vi "scripting build FXP VIs.vi"() -> ()   [LabVIEW 2020]
uses:
  <vilib>/numeric/LVNumericRepresentation.ctl
  <vilib>/Utility/traverseref.llb/TRef TravTarget.ctl
  <vilib>/Utility/traverseref.llb/VI Scripting - Traverse.lvlib
panel:
  out "error out 4":errorcluster
  out "Traverse All":string[][](table)
  out "error out 3":errorcluster
  in  "Array Ref.":refnum<vi>
  in  "Representation":T1(ring)
  in  "error in (no error)":errorcluster
  out "Ref. Out":refnum<vi>
  out "error out":errorcluster
  out "error out 2":errorcluster
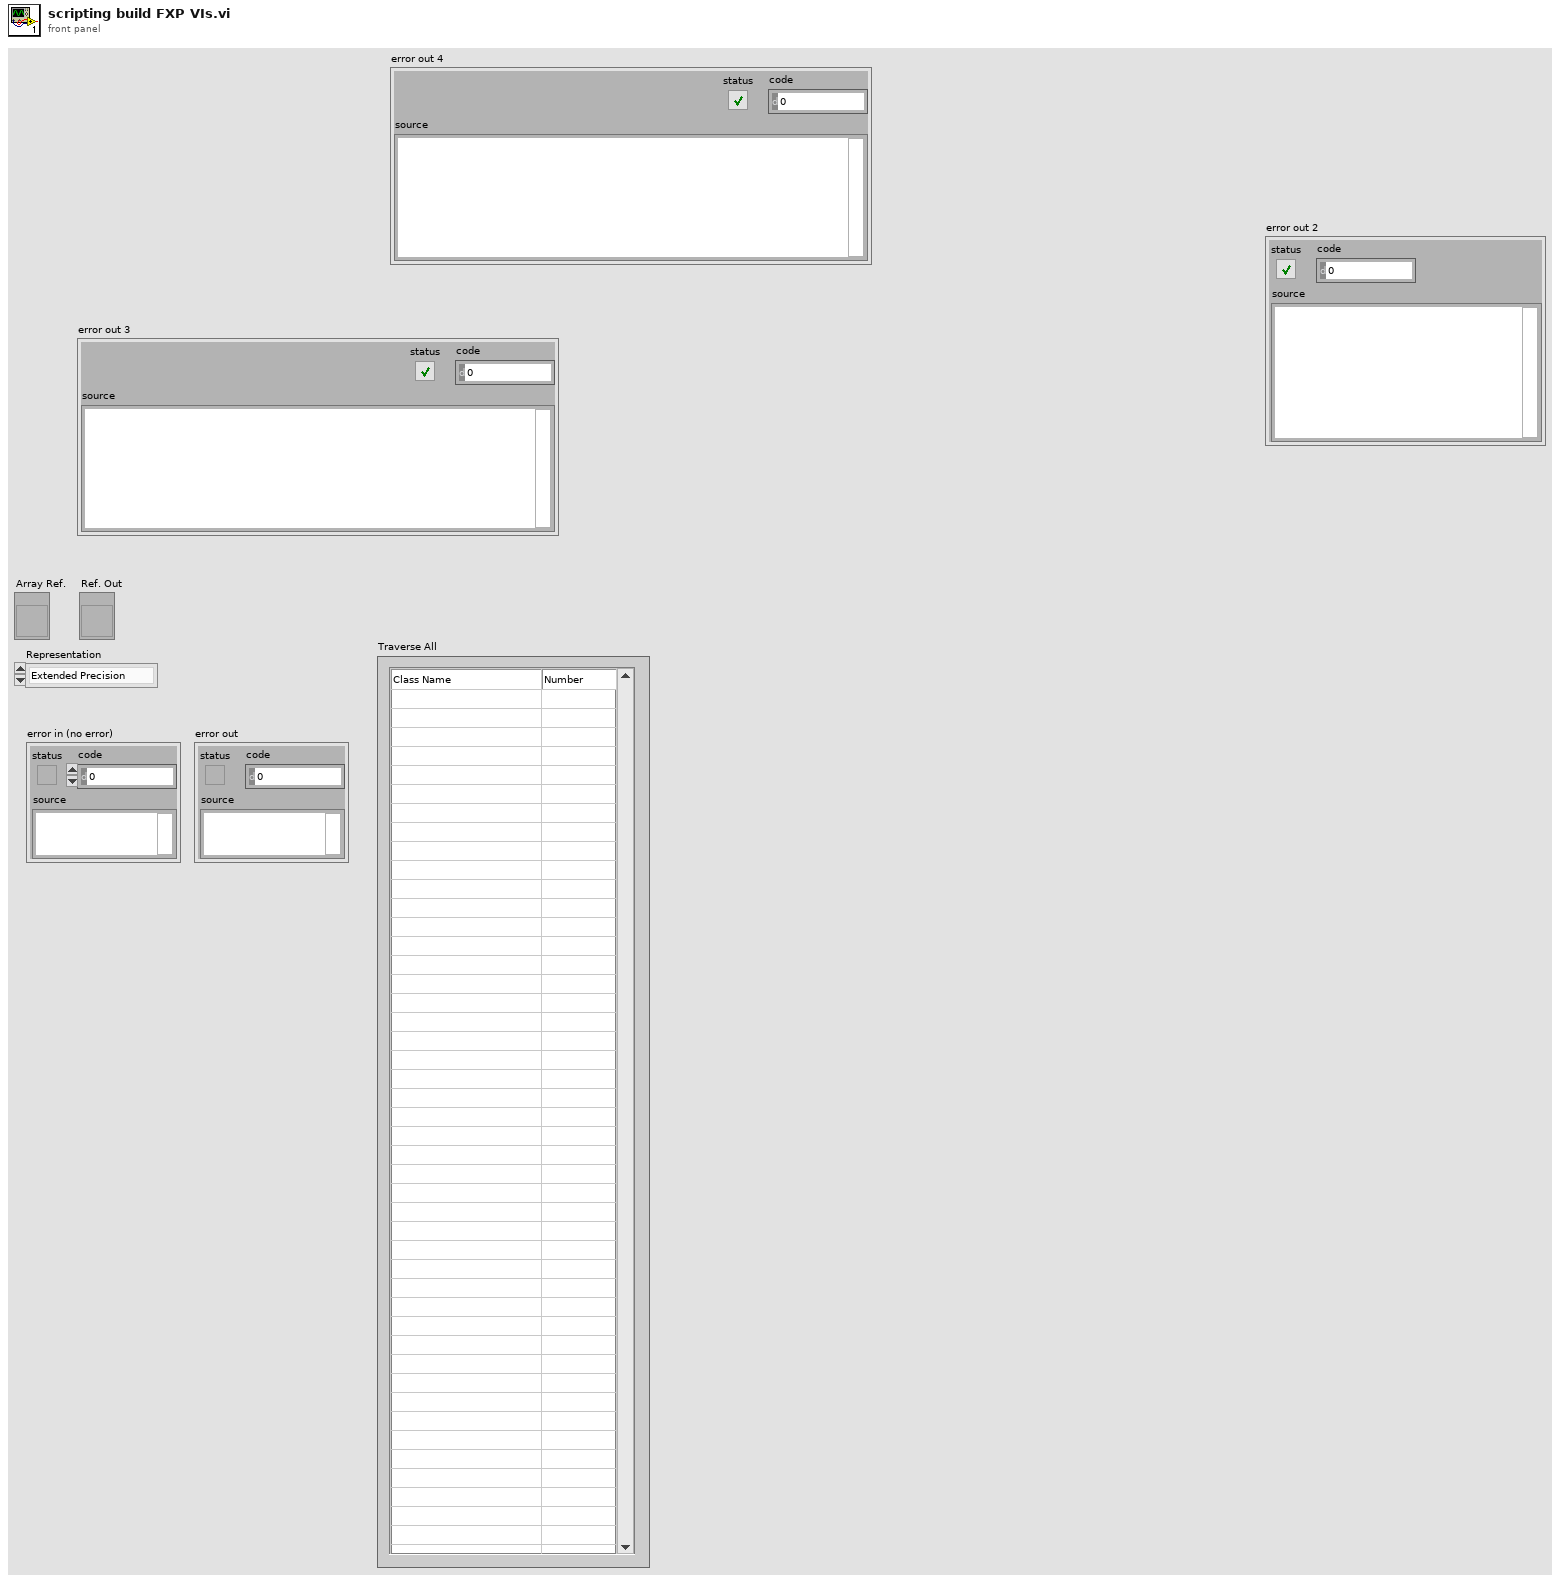
[diagram p1: front panel]
types:
  T1 = enum32{"Extended Precision", "Double Precision", "Single Precision", "Long", "Word", "Byte", "Unsigned Long", "Unsigned Word", "Unsigned Byte", "Complex Extended", "Complex Double", "Complex Single", "Quad", "Unsigned Quad", "Fixed-Point"}
  T2 = typedef "TRef TravTarget.ctl" = enum16{"FP", "BD", "Other"}
  T3 = typedef "LVNumericRepresentation.ctl" = enum32{"Extended Precision", "Double Precision", "Single Precision", "Long", "Word", "Byte", "Unsigned Long", "Unsigned Word", "Unsigned Byte", "Complex Extended", "Complex Double", "Complex Single", "Quad", "Unsigned Quad", "Fixed-Point"}
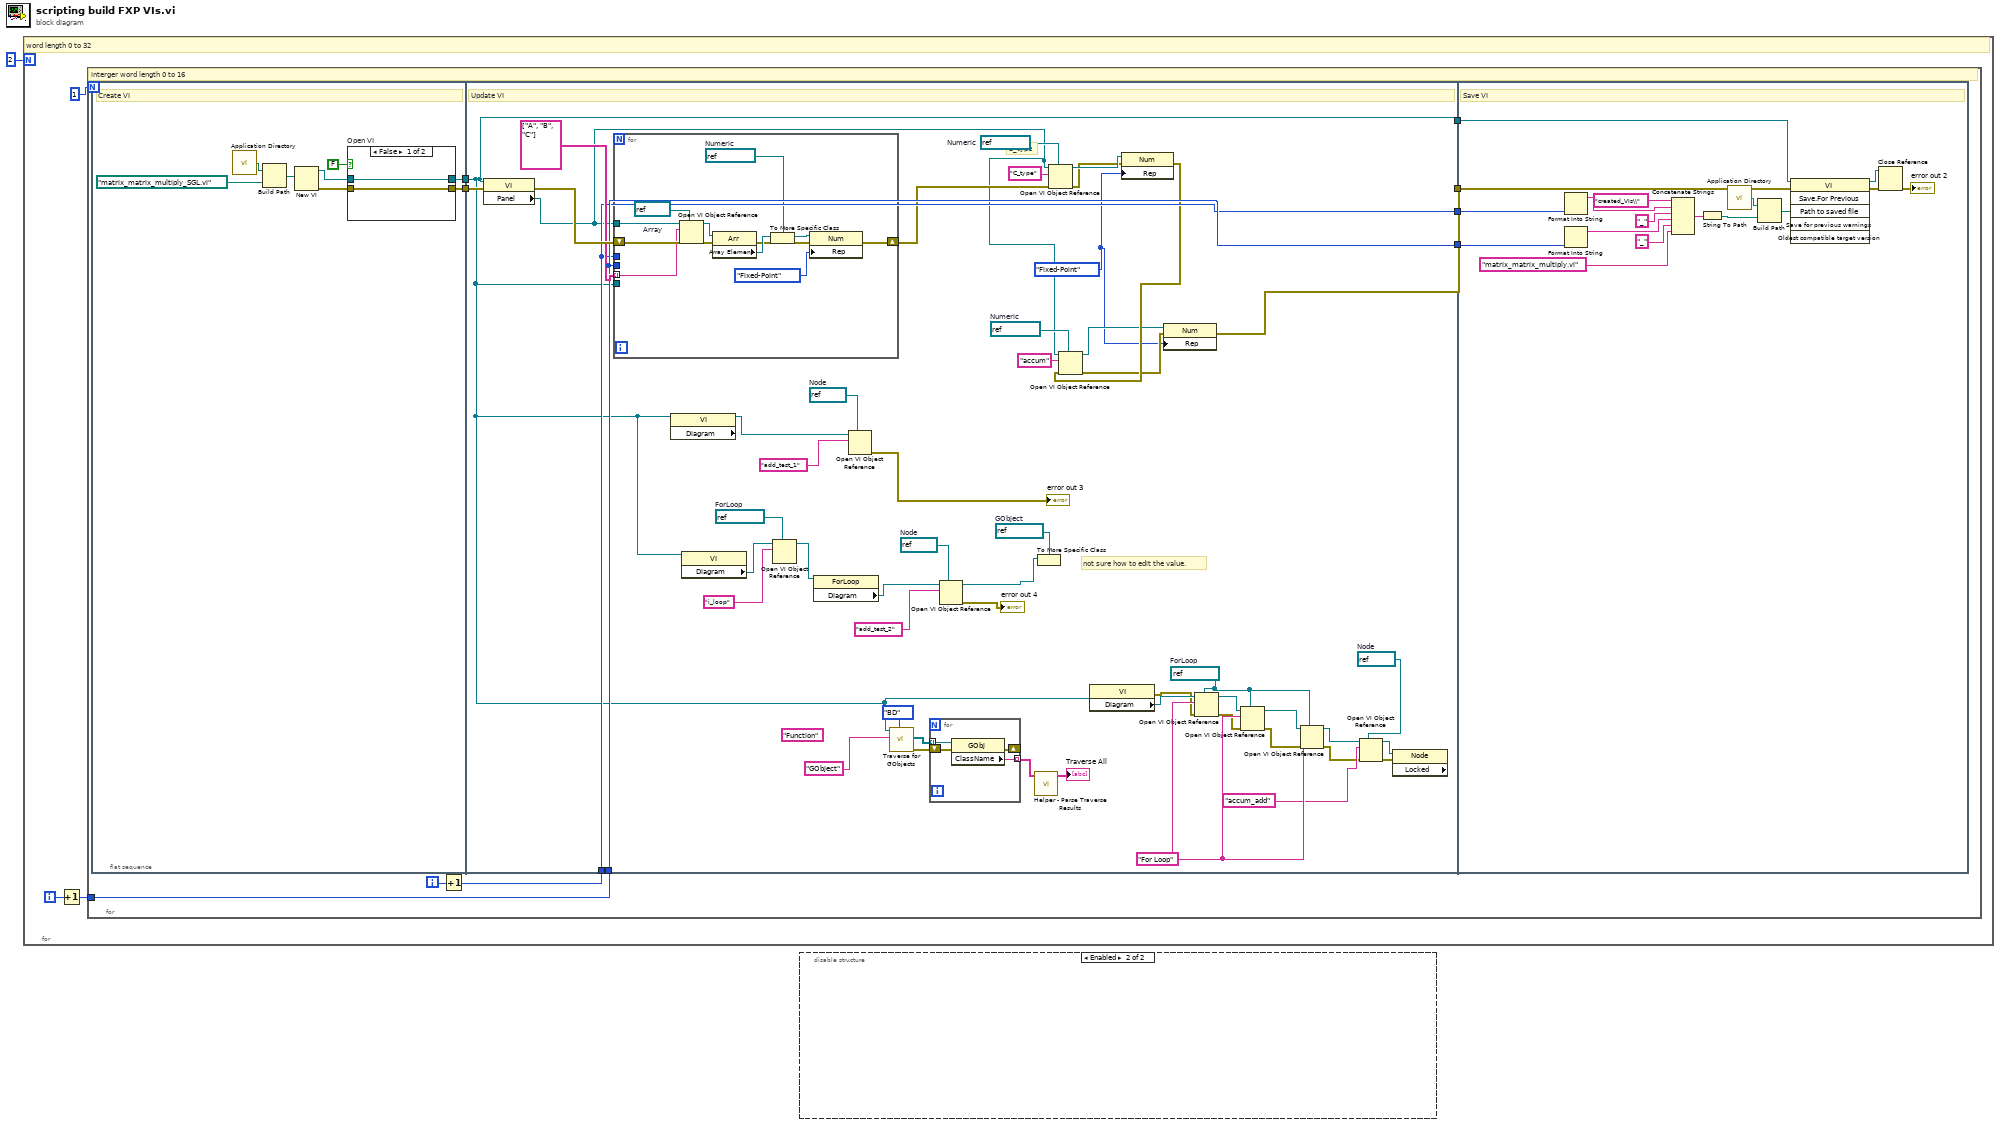
[diagram p0: block diagram]
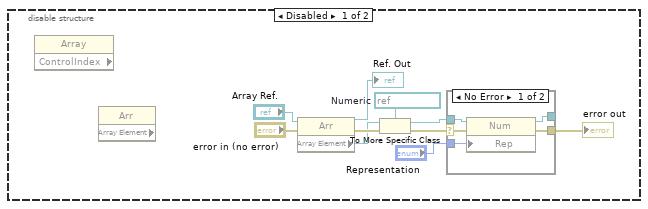
[diagram p2: hidden frame]
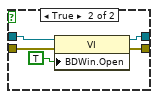
[diagram p4: hidden frame]
diagram:
  n1 = for {
    N: 2 -> [_]
    i -> [w4]
    # "word length 0 to 32"
    n2 = Increment(x=w4) -> (x+1=w2:i32)
    n3 = for {
      N: 1 -> [_]
      tunnel: w2 -> [w7]
      i -> [w6]
      # "interger word length 0 to 16"
      n4 = flat-sequence {
        tunnel: [w14] -> w13
        tunnel: [w15] -> w12
        tunnel: w5 -> [w77]
        tunnel: w7 -> [w78]
        tunnel: w13 -> [w35]
        tunnel: w12 -> [w79]
        tunnel: [w67] -> w11
        tunnel: [w78] -> w10
        tunnel: [w77] -> w9
        tunnel: [w35] -> w8
        tunnel: w11 -> [w103]
        tunnel: w10 -> [w101]
        tunnel: w9 -> [w100]
        tunnel: w8 -> [w99]
        frame #0 {
          # "Create VI"
          n5 = call <vilib>:"Application Directory.vi"() -> ("Application Directory"=w20:path)
          n6 = Build Path(base path=w20, name or relative path=path "matrix_matrix_multiply_SGL.vi" ("vi path")) -> (appended path=w21:path)
          n7 = New VI(10:w21) -> (0:w19:errorcluster, 3:w18:refnum<vi>)  [unwired: 6 in]
          n8 = case "Open VI" shown="False" FALSE {
            tunnel: w18 -> [w22 w28]
            tunnel: w19 -> [w23 w27]
            tunnel: [w22 w25] -> w14
            tunnel: [w23 w24] -> w15
            frame False {
            }
            frame True {
              n9 = property class="VI"(reference=w28, error in=w27, "BDWin.Open"=TRUE ("Block Diagram Window:Open")) -> (reference out=w25:refnum<vi>, error out=w24:errorcluster)
            }
          }
        }
        frame #1 {
          w29 = refnum<vi> refnum  # GObject
          w36 = refnum<vi> refnum  # ForLoop
          w40 = refnum<vi> refnum  # Node
          w49 = refnum<vi> refnum  # Node
          w50 = "For Loop" ("name/order")
          w51 = refnum<vi> refnum  # ForLoop
          (unwired) "Function"
          w63 = refnum<vi> refnum  # Node
          w71 = refnum<vi> refnum  # Numeric
          w64 = LVNumericRepresentation."Fixed-Point" ("Representation")
          w76 = refnum<vi> refnum  # Numeric
          # "not sure how to edit the value."
          # "C_type"
          # "Update VI"
          n10 = property on="Property Node" class="VI"(reference=w35, error in=w79) -> (error out=w81:errorcluster, "Panel"=w69:refnum<vi>)  [unwired: 1 out]
          n11 = for {
            tunnel: w69 -> [w95]
            tunnel: w77 -> [_]
            tunnel: w78 -> [_]
            shift-right: [w86] -> w74
            shift-left: w81 -> [w97]
            tunnel: string[] ["A", "B", "C"] -> [w96] mode=indexing
            tunnel: w35 -> [_]
            w93 = refnum<vi> refnum  # Numeric
            w98 = refnum<vi> refnum  # Array
            n12 = Open VI Object Reference(7:w98, 8:w97, 10:w96, 11:w95) -> (0:w89:errorcluster, 3:w90:refnum<vi>)
            n13 = property class="Arr"(reference=w90, error in=w89) -> (error out=w88:errorcluster, "Array Element"=w94:refnum<vi>)  [unwired: 1 out]
            n14 = To More Specific Class(target class=w93, reference=w94, error in=w88) -> (specific class reference=w92:refnum<vi>, error out=w87:errorcluster)
            n15 = property class="Num"(reference=w92, error in=w87, "Rep"=LVNumericRepresentation."Fixed-Point" ("Representation")) -> (error out=w86:errorcluster)  [unwired: 1 out]
          }
          n16 = property on="Property Node" class="VI" props=["Diagram"](reference=w35) -> (reference out=w33:refnum<vi>)  [unwired: 1 in, 2 out]
          n17 = property on="Property Node" class="VI"(reference=w35) -> ("Diagram"=w38:refnum<vi>)  [unwired: 1 in, 2 out]
          n18 = Open VI Object Reference(7:w36, 10:"i_loop" ("name/order"), 11:w38) -> (3:w32:refnum<vi>)  [unwired: 1 in, 1 out]
          n19 = property on="Property Node" class="ForLoop"(reference=w32) -> ("Diagram"=w31:refnum<vi>)  [unwired: 1 in, 2 out]
          n20 = Open VI Object Reference(7:w63, 10:"add_test_1" ("name/order"), 11:w33) -> (0:→"error out 3":errorcluster)  [unwired: 1 in, 1 out]
          n21 = call <vilib>:"Traverse for GObjects.vi"("Traverse Target"=TRef_TravTarget."BD", "Class Name"="GObject", "VI Refnum"=w35) -> ("error out"=w58:errorcluster, "References"=w59:refnum<vi>[])  [unwired: 5 in, 2 out]
          n22 = for {
            tunnel: w59 -> [w85] mode=indexing
            tunnel: [w84] -> w57 mode=indexing
            shift-right: [w82] -> _
            shift-left: w58 -> [w83]
            n23 = property class="GObj"(reference=w85, error in=w83) -> (error out=w82:errorcluster, "ClassName"=w84:string)  [unwired: 1 out]
          }
          n24 = Open VI Object Reference(7:w40, 10:"add_test_2" ("name/order"), 11:w31) -> (0:→"error out 4":errorcluster, 3:w30:refnum<vi>)  [unwired: 1 in]
          n25 = call "Helper - Parse Traverse Results.vi"("Traverse Results"=w57) -> ("Parsed Results"=→"Traverse All":string[][])  [unwired: 10 in]
          n26 = To More Specific Class(target class=w29, reference=w30) -> ()  [unwired: 1 in, 2 out]
          n27 = Open VI Object Reference(7:w76, 8:w74, 10:"C_type" ("name/order"), 11:w69) -> (0:w72:errorcluster, 3:w73:refnum<vi>)
          n28 = property on="Property Node" class="VI"(reference=w35) -> (error out=w46:errorcluster, "Diagram"=w54:refnum<vi>)  [unwired: 1 in, 1 out]
          n29 = property class="Num"(reference=w73, error in=w72, "Rep"=w64) -> (error out=w68:errorcluster)  [unwired: 1 out]
          n30 = Open VI Object Reference(7:w71, 8:w68, 10:"accum" ("name/order"), 11:w69) -> (0:w66:errorcluster, 3:w65:refnum<vi>)
          n31 = property class="Num"(reference=w65, error in=w66, "Rep"=w64) -> (error out=w67:errorcluster)  [unwired: 1 out]
          n32 = Open VI Object Reference(7:w51, 8:w46, 10:w50, 11:w54) -> (0:w45:errorcluster, 3:w52:refnum<vi>)
          n33 = Open VI Object Reference(7:w51, 8:w45, 10:w50, 11:w52) -> (0:w44:errorcluster, 3:w53:refnum<vi>)
          n34 = Open VI Object Reference(7:w51, 8:w44, 10:w50, 11:w53) -> (0:w43:errorcluster, 3:w48:refnum<vi>)
          n35 = Open VI Object Reference(7:w49, 8:w43, 10:"accum_add" ("name/order"), 11:w48) -> (0:w41:errorcluster, 3:w42:refnum<vi>)
          n36 = property class="Node" props=["Locked"](reference=w42, error in=w41) -> ()  [unwired: 3 out]
        }
        frame #2 {
          # "Save VI"
          n37 = Format Into String(w100) -> (resulting string=w113:string)  [unwired: 3 in, 1 out]
          n38 = Format Into String(w101) -> (resulting string=w114:string)  [unwired: 3 in, 1 out]
          n39 = Concatenate Strings("created_VIs\\" ("string"), w113, "_" ("string"), w114, "_" ("string"), "matrix_matrix_multiply.vi" ("string")) -> (w102:string)
          n40 = String To Path(string=w102) -> (path=w115:path)
          n41 = call <vilib>:"Application Directory.vi"() -> ("Application Directory"=w111:path)
          n42 = Build Path(base path=w111, name or relative path=w115) -> (appended path=w112:path)
          n43 = invoke class="VI" method="Save.For Previous"(reference=w99, error in=w103, "Path to saved file"=w112) -> (reference out=w108:refnum<vi>, error out=w109:errorcluster)  [unwired: 3 in, 4 out]
          n44 = Close Reference(reference=w108, error in (no error)=w109) -> (error out=→"error out 2":errorcluster)
        }
      }
      n45 = Increment(x=w6) -> (x+1=w5:i32)
    }
  }
  n46 = disable-structure shown="Enabled" {
    frame Disabled {
      w124 = refnum<vi> refnum  # Numeric
      n47 = property on="Property Node" class="Array" props=["ControlIndex"]() -> ()  [unwired: 2 in, 3 out]
      n48 = property class="Arr" props=["Array Element"]() -> ()  [unwired: 2 in, 3 out]
      n49 = property class="Arr"(reference="Array Ref.", error in="error in (no error)") -> (reference out=→"Ref. Out":refnum<vi>, error out=w119:errorcluster, "Array Element"=w116:refnum<vi>)
      n50 = To More Specific Class(target class=w124, reference=w116, error in=w119) -> (specific class reference=w122:refnum<vi>, error out=w123:errorcluster)
      n51 = case shown="No Error" w123 {
        selector: w123 -> [w130 _]
        tunnel: w122 -> [w129 w131]
        tunnel: "Representation" -> [w128 _]
        tunnel: [w127 w131] -> _
        tunnel: [w126 _] -> w117
        frame No Error {
          n52 = property class="Num"(reference=w129, error in=w130, "Rep"=w128) -> (reference out=w127:refnum<vi>, error out=w126:errorcluster)
        }
        frame Error {
        }
      }
      "error out" <- w117
    }
    frame Enabled {
    }
  }
